vi "Separate Array Values.vi"(0 "Input Array":dbl[](array[numeric])=[6.0, 3.9, -5.8, 0.0, -2.6, -1.0, 2.2, -4.3]) -> (1 "Positive Array":dbl[](array[numeric]), 2 "Negative Array":dbl[](array[numeric]))   [LabVIEW 2012]
doc: "This VI takes an input array that contains a mixture of positive and negative values and separates that array into two smaller arrays - one containing just the negative values and one containing just the positive values. \n\nConditional auto-indexing is used to separate the positive numbers from the negative numbers."
panel:
  # "This VI will sort the Input Array into two separate 1D arrays containing positive values and negative values."
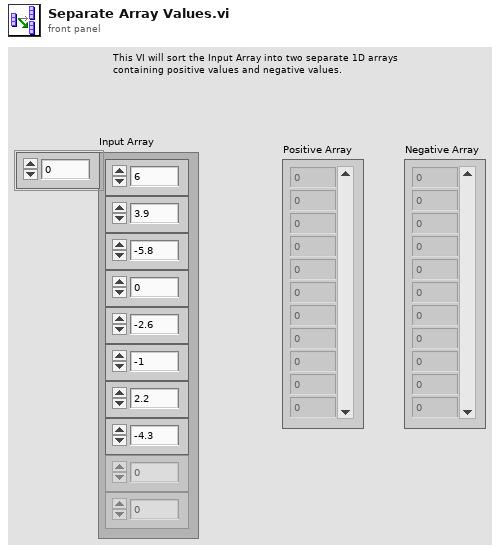
[diagram p1: front panel]
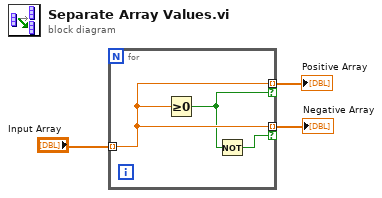
[diagram p0: block diagram]
diagram:
  n1 = for {
    tunnel: "Input Array" -> [w6] mode=indexing
    tunnel: [w6] -> w2 mode=indexing if=w5
    tunnel: [w6] -> w1 mode=indexing if=w4
    n2 = Greater Or Equal To 0?(x=w6) -> (x >= 0?=w5:bool)
    n3 = Not(x=w5) -> (.not. x?=w4:bool)
  }
  "Positive Array" <- w2
  "Negative Array" <- w1
